vi "Circuit.vi"() -> ()   [LabVIEW 2019]
uses:
  <vilib>/MakerHub/LINX/Public/Peripherals/Analog/Analog Read 1 Chan.vi
  <vilib>/MakerHub/LINX/Public/Peripherals/Analog/Analog Read N Chans.vi
  <vilib>/MakerHub/LINX/Private/Local IO/LinxAnalogRead.vi
  <vilib>/MakerHub/LINX/Public/Utilities/Check Channel.vi
  <vilib>/MakerHub/LINX/Public/Utilities/Open Serial.vi
  <vilib>/MakerHub/LINX/Private/Utilties/Generate Error.vi
  <vilib>/MakerHub/LINX/LMH-LINX.lvlib
panel:
  out "current time 3":timestamp
  in  "milliseconds to wait":u32
  in  "stop 2":bool
  out "current time 2":timestamp
  out "acc time":timestamp
  in  "Serial Port":refnum<visa-resource-name>="N/A"
  in  "y":dbl
  in  "stop":bool
  out "Voltage":dbl
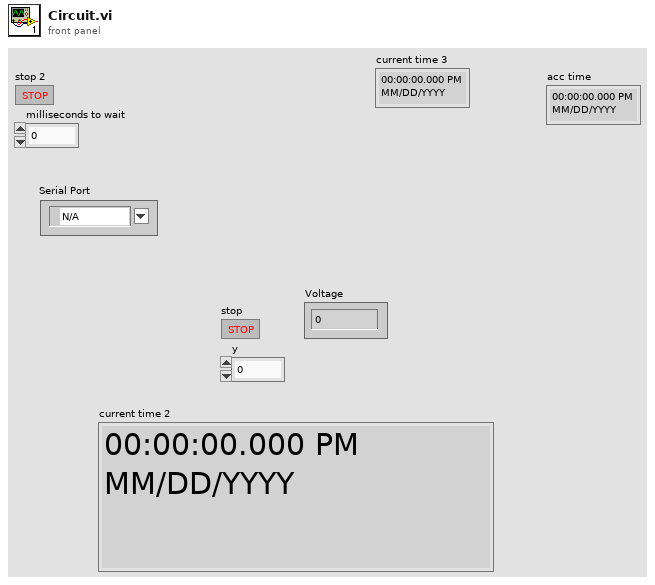
[diagram p1: front panel]
types:
  T1 = typedef "LMH-LINX.lvlib/LINX Ref.ctl" = cluster{"IO":T2, "Interface":T3, "LINX Device Config":T4}
  T2 = typedef "LMH-LINX.lvlib/Platform.ctl" = enum16{"Remote", "Local"}
  T3 = typedef "LMH-LINX.lvlib/Interface.ctl" = enum16{"Serial", "TCP"}
  T4 = typedef "LMH-LINX.lvlib/Device.lvlib/LINX Device Config.ctl" = cluster{"Interface":T3, "COM Port":refnum<visa-resource-name>, "TCP Configuration":T5, "Device Family":u8, "Device ID":u8, "Device Name":string, "TCP Ref":refnum<k5>, "Channels":T6}
  T5 = typedef "LMH-LINX.lvlib/Device.lvlib/TCP Config.ctl" = cluster{"IP Address":string, "Port":u16}
  T6 = typedef "LMH-LINX.lvlib/Channels.ctl" = cluster{"DI":u8[], "DO":u8[], "AI":u8[], "AO":u8[], "PWM":u8[], "QE":u8[], "UART":u8[], "I2C 2":u8[], "SPI":u8[], "CAN":u8[], "Servo":u8[], "AI Ref (V)":dbl, "AI Resolution (Bits)":u8, "AO Ref (V)":dbl, "AO Resolution (Bits)":u8}
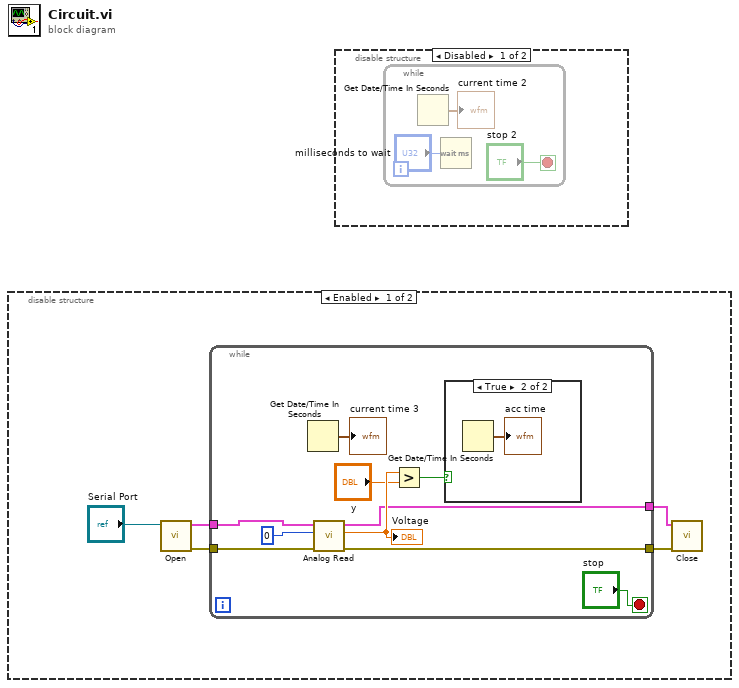
[diagram p0: block diagram]
diagram:
  n1 = disable-structure shown="Enabled" {
    frame Enabled {
      n2 = call-poly <vilib>:"Open.vi"("Serial Port"="Serial Port") -> ("Error Out"=w5:errorcluster, "LINX Resource"=w4:T1)  [unwired: 8 in, 1 out]
      n3 = while {
        tunnel: w5 -> [w11]
        tunnel: w4 -> [w10]
        tunnel: [w9] -> w3
        tunnel: [w8] -> w2
        stop <- "stop" stop-if-true
        n4 = Get Date/Time In Seconds() -> (seconds since 1Jan1904=→"current time 3":timestamp)
        n5 = call-poly <vilib>:"Analog Read.vi"("Error In"=w11, "Analog Channel"=u8 0, "LINX Resource"=w10) -> ("Error Out"=w9:errorcluster, "Voltage"=w13:dbl, "LINX Resource"=w8:T1)  [unwired: 5 in, 1 out]
        "Voltage" <- w13
        n6 = Greater?(x=w13, y="y") -> (0:w7:bool)
        n7 = case shown="True" w7 {
          frame False {
          }
          frame True {
            n8 = Get Date/Time In Seconds() -> (seconds since 1Jan1904=→"acc time":timestamp)
          }
        }
      }
      n9 = call <vilib>:"Close.vi"("Error In"=w3, "LINX Resource"=w2) -> ()  [unwired: 9 in, 1 out]
    }
    frame Disabled {
    }
  }
  n10 = disable-structure shown="Disabled" {
    frame Disabled {
      n11 = while {
        stop <- "stop 2" stop-if-true
        n12 = Get Date/Time In Seconds() -> (seconds since 1Jan1904=→"current time 2":timestamp)
        n13 = Wait (ms)(milliseconds to wait="milliseconds to wait") -> ()  [unwired: 1 out]
      }
    }
    frame Enabled {
    }
  }
